vi "Check if File or Folder Exists.vi"(8 "error in (no error)":errorcluster, 11 "path":path) -> (0 "error out":errorcluster, 2 "file or folder exists?":bool, 3 "dup path":path)   [LabVIEW 2010]
doc: "Checks whether a file or folder exists on disk at a specified path. This VI works with standard files and folders as well as files in LLB files."
uses:
  <vilib>/Utility/lvfile.llb/FT_FileTypes.ctl
  <vilib>/Utility/lvfile.llb/NI_FileType.lvlib
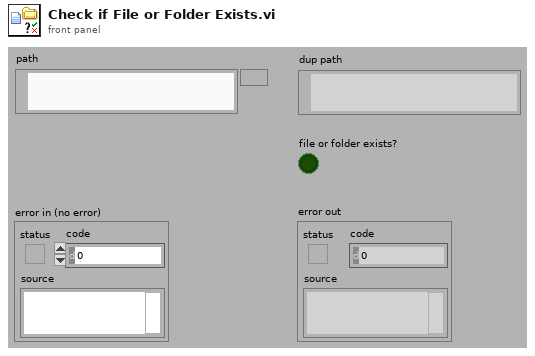
[diagram p1: front panel]
types:
  T1 = typedef "NI_FileType.lvlib/FT_FileTypes.ctl" = enum32{"Invalid file/path", "Unknown type", "Instrument", "Control", "Polymorphic VI", "Project", "Library", "LVClass", "XControl", "XNode", "CIN", "Run-time menu", "Palette menu", "LLB", "Shortcut", "Directory", "Class Private Data Control", "Statechart", "MathScript .m file", "Ladder Diagram", "LVLibp"}
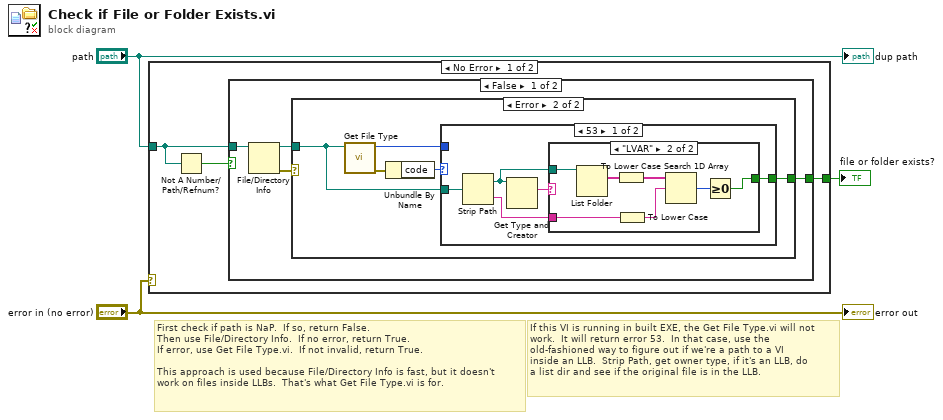
[diagram p0: block diagram]
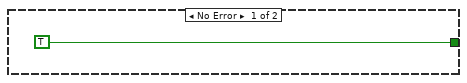
[diagram p2: hidden frame]
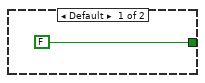
[diagram p3: hidden frame]
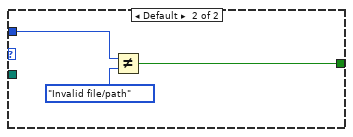
[diagram p4: hidden frame]
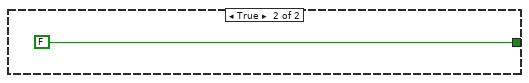
[diagram p5: hidden frame]
diagram:
  # "If this VI is running in built EXE, the Get File Type.vi will not\nwork.  It will return error 53.  In that case, use the\nold-fashioned way to figure out if we're a path to a VI\ninside an LLB.  Strip Path, get owner type, if it's an LLB, do\na list dir and see if the original file is in the LLB."
  # "First check if path is NaP.  If so, return False.\nThen use File/Directory Info.  If no error, return True.\nIf error, use Get File Type.vi.  If not invalid, return True.\n\nThis approach is used because File/Directory Info is fast, but it doesn't\nwork on files inside LLBs.  That's what Get File Type.vi is for."
  n1 = case shown="No Error" "error in (no error)" {
    tunnel: "path" -> [w5 _]
    tunnel: [w6 _] -> w1
    frame No Error {
      n2 = Not A Number/Path/Refnum?(number/path/refnum=w5) -> (NaN/Path/Refnum?=w4:bool)
      n3 = case shown="False" w4 {
        tunnel: [w8 FALSE] -> w6
        tunnel: w5 -> [w10 _]
        frame False {
          n4 = File/Directory Info(path=w10) -> (path out=w7:path, error out=w9:errorcluster)  [unwired: 1 in, 5 out]
          n5 = case shown="Error" w9 {
            tunnel: [TRUE w16] -> w8
            tunnel: w7 -> [_ w12]
            frame No Error {
            }
            frame Error {
              n6 = call <vilib>:"Get File Type.vi"("path"=w12) -> ("error out"=w14:errorcluster, "file type"=w15:T1)  [unwired: 1 in, 8 out]
              n7 = Unbundle By Name(w14) -> ("code"=w13:i32)
              n8 = case shown="53" w13 {
                tunnel: [w19 w32] -> w16
                tunnel: w15 -> [_ w31]
                tunnel: w12 -> [w21 _]
                frame 53 {
                  n9 = Strip Path(path=w21) -> (stripped path=w17:path, name=w18:string)
                  n10 = Get Type and Creator(7:w17) -> (2:w20:string)  [unwired: 1 in, 3 out]
                  n11 = case shown="\"LVAR\"" w20 {
                    tunnel: [FALSE w23] -> w19
                    tunnel: w18 -> [_ w27]
                    tunnel: w17 -> [_ w29]
                    frame Default {
                    }
                    frame "LVAR" {
                      n12 = List Folder(path=w29) -> (filenames=w28:string[])  [unwired: 1 in, 5 out]
                      n13 = To Lower Case(string=w28) -> (all lower case string=w25:string[])
                      n14 = To Lower Case(string=w27) -> (all lower case string=w26:string)
                      n15 = Search 1D Array(1D array=w25, element=w26) -> (index of element=w24:i32)  [unwired: 1 out]
                      n16 = Greater Or Equal To 0?(x=w24) -> (x >= 0?=w23:bool)
                    }
                  }
                }
                frame Default {
                  n17 = Not Equal?(x=w31, y=FT_FileTypes."Invalid file/path") -> (x != y?=w32:bool)
                }
              }
            }
          }
        }
        frame True {
        }
      }
    }
    frame Error {
    }
  }
  "file or folder exists?" <- w1
  "error out" <- "error in (no error)"
  "dup path" <- "path"
